vi "SetOutputVoltage.vi"(6 "Error In":errorcluster, 8 "channel(1,2)":string="1", 9 "Voltage":dbl, 10 "V_pre":dbl, 11 "Keithley 6482":refnum<visa-resource-name>) -> (0 "Error Out":errorcluster, 3 "Keithley 6483":refnum<visa-resource-name>)   [LabVIEW 2010, in "Keithley-6482-Visa.lvlib"]
uses:
  <instrlib>/lib-labview-8.6-export/Keithley-6482-Visa.lvlib
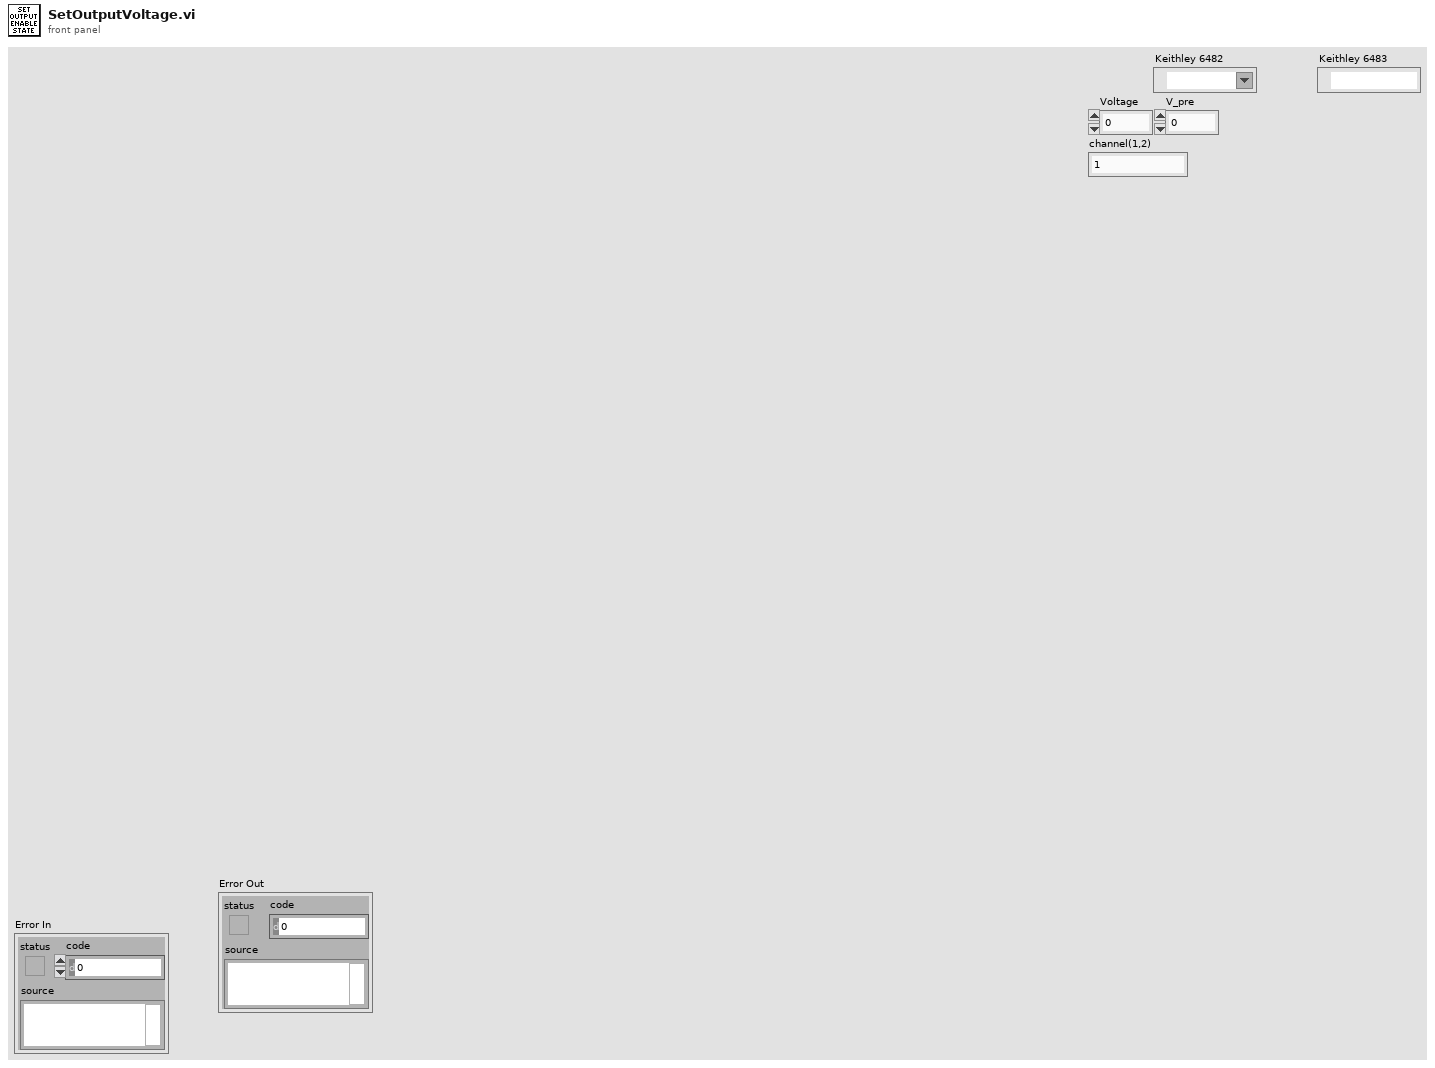
[diagram p1: front panel]
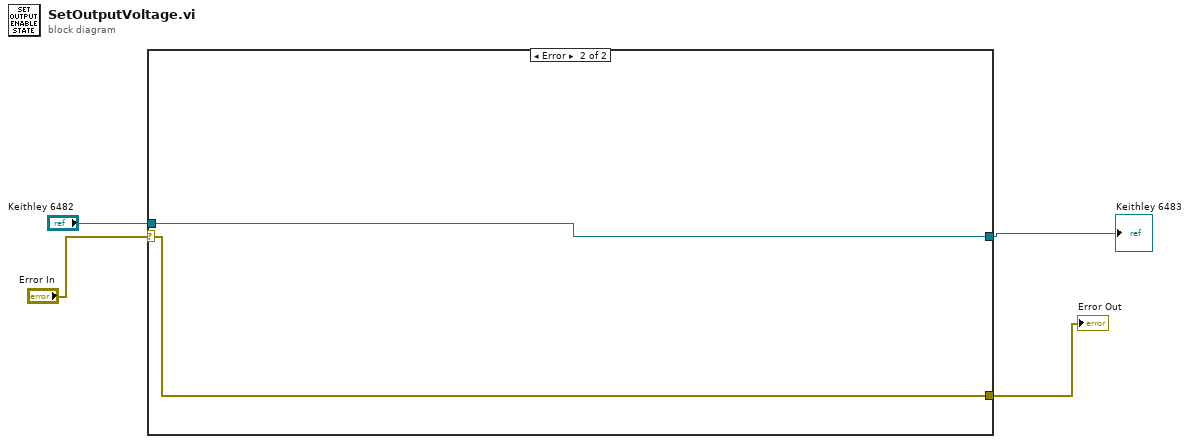
[diagram p0: block diagram]
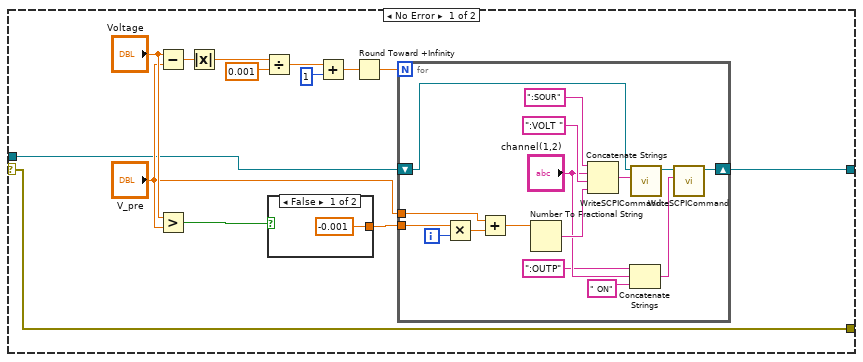
[diagram p2: hidden frame]
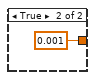
[diagram p3: hidden frame]
diagram:
  n1 = case shown="Error" "Error In" {
    selector: "Error In" -> [w5 w38]
    tunnel: "Keithley 6482" -> [w7 w37]
    tunnel: [w6 w37] -> w3
    tunnel: [w5 w38] -> w1
    frame No Error {
      n2 = Subtract(x="Voltage", y="V_pre") -> (x-y=w16:dbl)
      n3 = Greater?(x="Voltage", y="V_pre") -> (0:w18:bool)
      n4 = Absolute Value(x=w16) -> (abs(x)=w15:dbl)
      n5 = Divide(x=w15, y=0.001) -> (x/y=w13:dbl)
      n6 = case shown="False" w18 {
        tunnel: [-0.001 ("Vstep") 0.001 ("Vstep")] -> w17
        frame False {
        }
        frame True {
        }
      }
      n7 = Add(x=w13, y=1) -> (x+y=w11:dbl)
      n8 = Round Toward +Infinity(x=w11) -> (ceil(x): smallest int >= x=w8:dbl)
      n9 = for {
        N: w8 -> [_]
        tunnel: "V_pre" -> [w31]
        tunnel: w17 -> [w26]
        shift-right: [w23] -> w6
        shift-left: w7 -> [w28]
        i -> [w27]
        n10 = Multiply(x=w26, y=w27) -> (x*y=w25:dbl)
        n11 = Add(x=w31, y=w25) -> (x+y=w30:dbl)
        n12 = Number To Fractional String(number=w30) -> (F-format string=w29:string)  [unwired: 3 in]
        n13 = Concatenate Strings(":SOUR", "channel(1,2)", ":VOLT ", w29) -> (w32:string)
        n14 = Concatenate Strings(":OUTP", "channel(1,2)", " ON") -> (w19:string)
        n15 = call <instrlib>:"WriteSCPICommand.vi"("SCPI Command"=w32, "Keithley 6482 In"=w28) -> ("Keithley 6482 Out"=w24:refnum<visa-resource-name>)  [unwired: 8 in, 1 out]
        n16 = call <instrlib>:"WriteSCPICommand.vi"("SCPI Command"=w19, "Keithley 6482 In"=w24) -> ("Keithley 6482 Out"=w23:refnum<visa-resource-name>)  [unwired: 8 in, 1 out]
      }
    }
    frame Error {
    }
  }
  "Keithley 6483" <- w3
  "Error Out" <- w1
